vi "build calibration image.vi"(0 "1-sided cal image":dbl[][](array[numeric])) -> (2 "2-sided cal image":dbl[][](array[numeric]), 3 "avg power spectrum of stack":dbl[](array[numeric]))   [LabVIEW 2014]
uses:
  <vilib>/Analysis/2dsp.llb/Power Spectrum (DBL).vi
  <vilib>/Analysis/NI_AALPro.lvlib
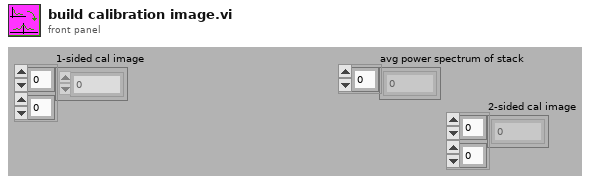
[diagram p1: front panel]
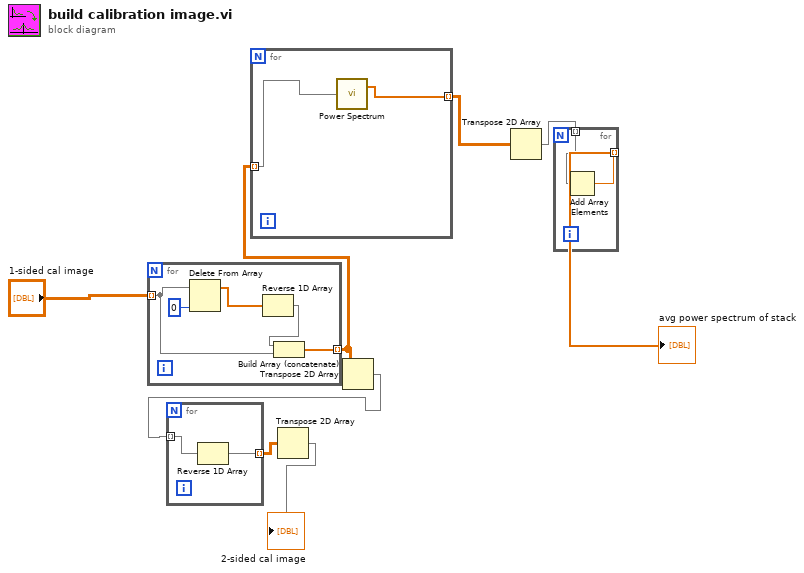
[diagram p0: block diagram]
diagram:
  n1 = for {
    tunnel: "1-sided cal image" -> [w10] mode=indexing
    tunnel: [w9] -> w6 mode=indexing
    n2 = Delete From Array(array=w10, index=0) -> (array with subset deleted=w12:dbl[])  [unwired: 1 in, 1 out]
    n3 = Reverse 1D Array(array=w12) -> (reversed array=w11:dbl[])
    n4 = Build Array (concatenate)(w11, w10) -> (w9:dbl[])
  }
  n5 = for {
    tunnel: w6 -> [w15] mode=indexing
    tunnel: [w14] -> w2 mode=indexing
    n6 = call-poly <vilib>:"Power Spectrum.vi"("X"=w15) -> ("Power Spectrum"=w14:dbl[])  [unwired: 1 out]
  }
  n7 = Transpose 2D Array(2D array=w6) -> (transposed array=w8:dbl[][])
  n8 = for {
    tunnel: w8 -> [w17] mode=indexing
    tunnel: [w16] -> w7 mode=indexing
    n9 = Reverse 1D Array(array=w17) -> (reversed array=w16:dbl[])
  }
  n10 = Transpose 2D Array(2D array=w7) -> (transposed array=→"2-sided cal image":dbl[][])
  n11 = Transpose 2D Array(2D array=w2) -> (transposed array=w5:dbl[][])
  n12 = for {
    tunnel: w5 -> [w19] mode=indexing
    tunnel: [w18] -> w4 mode=indexing
    n13 = Add Array Elements(numeric array=w19) -> (sum=w18:dbl)
  }
  "avg power spectrum of stack" <- w4
